vi "NiSwitch SetAttributeViReal64.vi"(6 "contextId":T1, 8 "error in":errorcluster, 9 "timeout (ms)":i32=-1, 10 "Request Data":T3, 11 "gRPC ID":T1) -> (0 "error out":errorcluster, 2 "Response Data":T2, 3 "gRPC ID out":T1)   [LabVIEW 2021, in "NI Switch_client.lvlib"]
uses:
  NI Switch_client.lvlib
  <vilib>/gRPC/LabVIEW gRPC Library/Shared/grpcId.ctl
  RPC Messages/niswitch_grpc_SetAttributeViReal64Request.ctl
  RPC Messages/nidevice_grpc_Session.ctl
  RPC Messages/niswitch_grpc_NiSwitchAttribute.ctl
  RPC Messages/niswitch_grpc_SetAttributeViReal64Response.ctl
  RPC Messages/niswitch_grpc_SetAttributeViReal64Response_Flat.ctl
  14035477-4c25-4107-8ed5-d0c4ef420ce5.vi
  RPC Messages/RichToFlatnidevice_grpc_Session.vi
  <vilib>/gRPC/LabVIEW gRPC Library/Shared/TranslateGrpcError.vi
  <vilib>/gRPC/LabVIEW gRPC Library/Shared/Wait On Occurrence Wrapper.vi
  <vilib>/gRPC/LabVIEW gRPC Library/Shared/Wait On Occurence.vi
  <vilib>/gRPC/LabVIEW gRPC Library/Server API/Server/Get Server DLL Path.vi
  <vilib>/Utility/error.llb/Error Cluster From Error Code.vi
  <vilib>/Utility/config.llb/Open Config Data.vi
  <vilib>/Utility/config.llb/Write Key.vi
  <vilib>/Utility/config.llb/Write Key (Boolean).vi
  <vilib>/Utility/config.llb/Not A Config Data Refnum.vi
  <vilib>/Utility/config.llb/Read Key.vi
  <vilib>/Utility/config.llb/Read Key (Boolean).vi
  <vilib>/Utility/config.llb/Close Config Data.vi
  <vilib>/gRPC/LabVIEW gRPC Library/grpc-lvsupport-release.lvlib
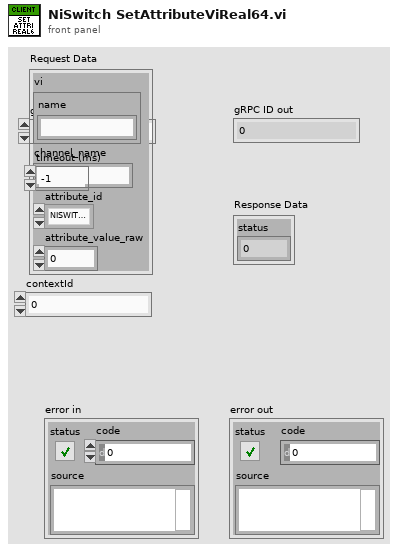
[diagram p1: front panel]
types:
  T1 = typedef "grpc-lvsupport-release.lvlib/grpcId.ctl" = u64
  T2 = typedef "NI Switch_client.lvlib/niswitch_grpc_SetAttributeViReal64Response.ctl" = cluster{"status":i32}
  T3 = typedef "NI Switch_client.lvlib/niswitch_grpc_SetAttributeViReal64Request.ctl" = cluster{"vi":T4, "channel_name":string, "attribute_id":T5, "attribute_value_raw":dbl}
  T4 = typedef "NI Switch_client.lvlib/nidevice_grpc_Session.ctl" = cluster{"name":string}
  T5 = typedef "NI Switch_client.lvlib/niswitch_grpc_NiSwitchAttribute.ctl" = enum32{"NISWITCH_ATTRIBUTE_UNSPECIFIED", "NISWITCH_ATTRIBUTE_RANGE_CHECK", "NISWITCH_ATTRIBUTE_QUERY_INSTRUMENT_STATUS", "NISWITCH_ATTRIBUTE_CACHE", "NISWITCH_ATTRIBUTE_SIMULATE", "NISWITCH_ATTRIBUTE_RECORD_COERCIONS", "NISWITCH_ATTRIBUTE_DRIVER_SETUP", "NISWITCH_ATTRIBUTE_INTERCHANGE_CHECK", "NISWITCH_ATTRIBUTE_CHANNEL_COUNT", "NISWITCH_ATTRIBUTE_SPECIFIC_DRIVER_PREFIX", "NISWITCH_ATTRIBUTE_IO_RESOURCE_DESCRIPTOR", "NISWITCH_ATTRIBUTE_LOGICAL_NAME", "NISWITCH_ATTRIBUTE_SUPPORTED_INSTRUMENT_MODELS", "NISWITCH_ATTRIBUTE_GROUP_CAPABILITIES", "NISWITCH_ATTRIBUTE_INSTRUMENT_FIRMWARE_REVISION", "NISWITCH_ATTRIBUTE_INSTRUMENT_MANUFACTURER", "NISWITCH_ATTRIBUTE_INSTRUMENT_MODEL", "NISWITCH_ATTRIBUTE_SPECIFIC_DRIVER_VENDOR", "NISWITCH_ATTRIBUTE_SPECIFIC_DRIVER_DESCRIPTION", "NISWITCH_ATTRIBUTE_SPECIFIC_DRIVER_CLASS_SPEC_MAJOR_VERSION", "NISWITCH_ATTRIBUTE_SPECIFIC_DRIVER_CLASS_SPEC_MINOR_VERSION", "NISWITCH_ATTRIBUTE_SPECIFIC_DRIVER_REVISION", "NISWITCH_ATTRIBUTE_SERIAL_NUMBER_I32", "NISWITCH_ATTRIBUTE_IS_WAITING_FOR_TRIG", "NISWITCH_ATTRIBUTE_TRIGGER_MODE", "NISWITCH_ATTRIBUTE_MASTER_SLAVE_TRIGGER_BUS", "NISWITCH_ATTRIBUTE_MASTER_SLAVE_SCAN_ADVANCED_BUS", "NISWITCH_ATTRIBUTE_CABLED_MODULE_TRIGGER_BUS", "NISWITCH_ATTRIBUTE_CABLED_MODULE_SCAN_ADVANCED_BUS", "NISWITCH_ATTRIBUTE_TRIGGER_INPUT_POLARITY", "NISWITCH_ATTRIBUTE_SCAN_ADVANCED_POLARITY", "NISWITCH_ATTRIBUTE_PARSED_SCAN_LIST", "NISWITCH_ATTRIBUTE_HANDSHAKING_INITIATION", "NISWITCH_ATTRIBUTE_NUMBER_OF_RELAYS", "NISWITCH_ATTRIBUTE_SERIAL_NUMBER", "NISWITCH_ATTRIBUTE_DIGITAL_FILTER_ENABLE", "NISWITCH_ATTRIBUTE_POWER_DOWN_LATCHING_RELAYS_AFTER_DEBOUNCE", "NISWITCH_ATTRIBUTE_ANALOG_BUS_SHARING_ENABLE", "NISWITCH_ATTRIBUTE_TEMPERATURE", "NISWITCH_ATTRIBUTE_IS_SOURCE_CHANNEL", "NISWITCH_ATTRIBUTE_IS_DEBOUNCED", "NISWITCH_ATTRIBUTE_IS_CONFIGURATION_CHANNEL", "NISWITCH_ATTRIBUTE_SETTLING_TIME", "NISWITCH_ATTRIBUTE_BANDWIDTH", "NISWITCH_ATTRIBUTE_MAX_DC_VOLTAGE", "NISWITCH_ATTRIBUTE_MAX_AC_VOLTAGE", "NISWITCH_ATTRIBUTE_MAX_SWITCHING_DC_CURRENT", "NISWITCH_ATTRIBUTE_MAX_SWITCHING_AC_CURRENT", "NISWITCH_ATTRIBUTE_MAX_CARRY_DC_CURRENT", "NISWITCH_ATTRIBUTE_MAX_CARRY_AC_CURRENT", "NISWITCH_ATTRIBUTE_MAX_SWITCHING_DC_POWER", "NISWITCH_ATTRIBUTE_MAX_SWITCHING_AC_POWER", "NISWITCH_ATTRIBUTE_MAX_CARRY_DC_POWER", "NISWITCH_ATTRIBUTE_MAX_CARRY_AC_POWER", "NISWITCH_ATTRIBUTE_CHARACTERISTIC_IMPEDANCE", "NISWITCH_ATTRIBUTE_WIRE_MODE", "NISWITCH_ATTRIBUTE_NUM_OF_ROWS", "NISWITCH_ATTRIBUTE_NUM_OF_COLUMNS", "NISWITCH_ATTRIBUTE_SCAN_LIST", "NISWITCH_ATTRIBUTE_SCAN_MODE", "NISWITCH_ATTRIBUTE_TRIGGER_INPUT", "NISWITCH_ATTRIBUTE_SCAN_ADVANCED_OUTPUT", "NISWITCH_ATTRIBUTE_IS_SCANNING", "NISWITCH_ATTRIBUTE_SCAN_DELAY", "NISWITCH_ATTRIBUTE_CONTINUOUS_SCAN"}
  T6 = typedef "NI Switch_client.lvlib/niswitch_grpc_SetAttributeViReal64Response_Flat.ctl" = cluster{"status":i32}
  T7 = typedef "NI Switch_client.lvlib/niswitch_grpc_SetAttributeViReal64Request_Flat.ctl" = cluster{"vi":T8, "channel_name":string, "attribute_id":T5, "attribute_value_raw":dbl}
  T8 = typedef "NI Switch_client.lvlib/nidevice_grpc_Session_Flat.ctl" = cluster{"name":string}
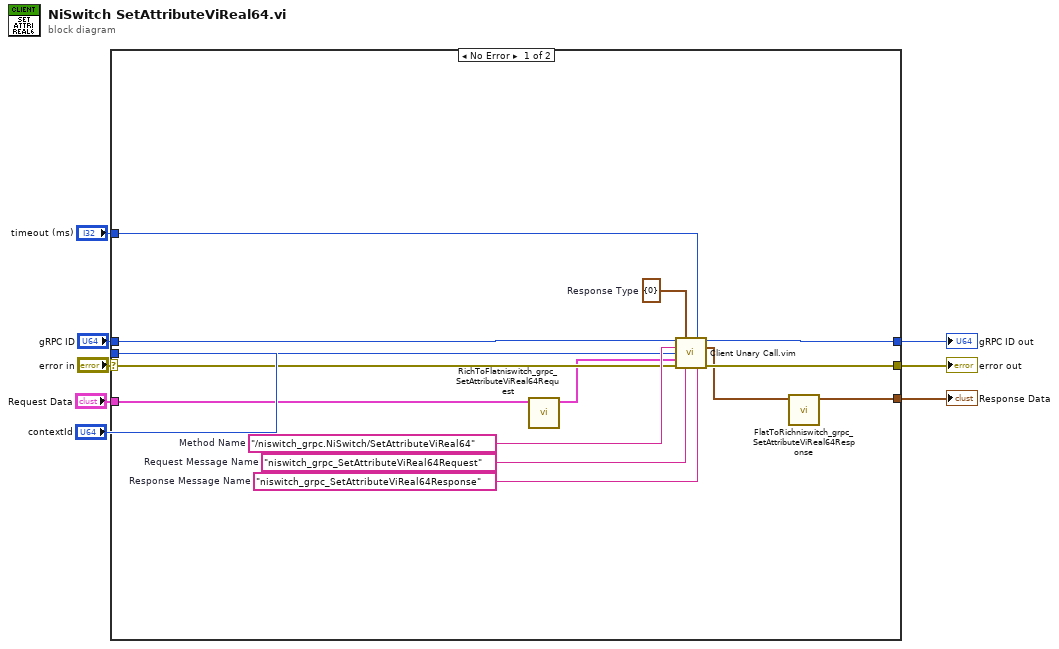
[diagram p0: block diagram]
diagram:
  n1 = case shown="No Error" "error in" {
    selector: "error in" -> [w18 w23]
    tunnel: [w17 w23] -> w7
    tunnel: "gRPC ID" -> [w16 w24]
    tunnel: [w15 w24] -> w5
    tunnel: "Request Data" -> [w12 _]
    tunnel: [w9 _] -> w3
    tunnel: "timeout (ms)" -> [w14 _]
    tunnel: "contextId" -> [w13 _]
    frame No Error {
      w19 = "niswitch_grpc_SetAttributeViReal64Response"  # Response Message Name
      w20 = "niswitch_grpc_SetAttributeViReal64Request"  # Request Message Name
      w21 = T6 {"status"=0}  # Response Type
      w22 = "/niswitch_grpc.NiSwitch/SetAttributeViReal64"  # Method Name
      n2 = call "RichToFlatniswitch_grpc_SetAttributeViReal64Request.vi"("InputCluster"=w12) -> ("OutputCluster"=w11:T7)  [unwired: 10 in]
      n3 = call "Client Unary Call.vim"("ClientID in"=w16, "Response Type"=w21, "timeout (ms)"=w14, "Method Name"=w22, "contextId"=w13, "Request Data"=w11, "error in"=w18, "Request Message Name"=w20, "Response Message Name"=w19) -> ("ClientID out"=w15:u64, "Response Data"=w10:T6, "error out"=w17:errorcluster)  [unwired: 4 in]
      n4 = call "FlatToRichniswitch_grpc_SetAttributeViReal64Response.vi"("InputCluster"=w10) -> ("OutputCluster"=w9:T2)  [unwired: 10 in]
    }
    frame Error {
    }
  }
  "error out" <- w7
  "gRPC ID out" <- w5
  "Response Data" <- w3
